vi "AILimits.vi"(0 "HighLimit":i16[](array[numeric])=[0, 0, 0, 0, 0, 0, 0, 0, 0, 0, 0, 0, 0, 0, 0, 0], 1 "ClearLimits":bool, 5 "LowLimit":i16[](array[numeric])=[0, 0, 0, 0, 0, 0, 0, 0, 0, 0, 0, 0, 0, 0, 0, 0], 7 "UnscaledAI":i16[](array[numeric])=[0, 0, 0, 0, 0, 0, 0, 0, 0, 0, 0, 0, 0, 0, 0, 0], 11 "index":i16, 12 "LimitsEnabled":u16 format="%.0x") -> (4 "UnscaledLimitLowOut":u16 format="%.0x", 6 "UnscaledLimitHighOut":u16 format="%.0x")   [LabVIEW 2017, in "ScaleAndLimit.lvlib"]
uses:
  ScaleAndLimit.lvlib
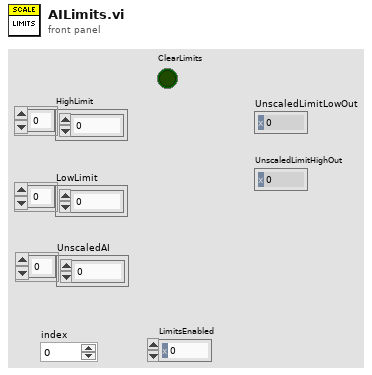
[diagram p1: front panel]
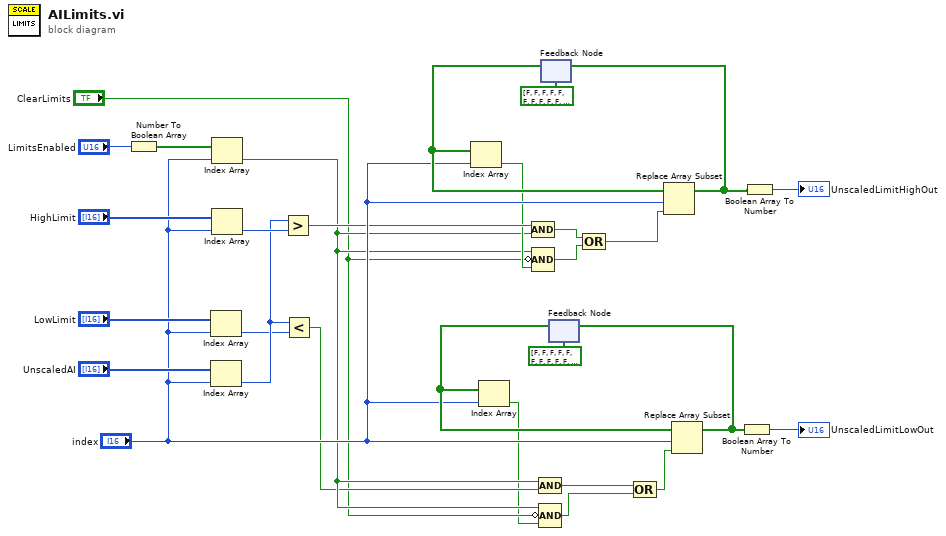
[diagram p0: block diagram]
diagram:
  n1 = Number To Boolean Array(number="LimitsEnabled") -> (Boolean array=w22:bool[])
  n2 = Index Array(array="LowLimit", index="index") -> (element=w24:i16)
  n3 = Index Array(array="UnscaledAI", index="index") -> (element=w25:i16)
  n4 = Index Array(array=w22, index="index") -> (element=w6:bool)
  n5 = Index Array(array="HighLimit", index="index") -> (element=w26:i16)
  n6 = Greater?(x=w25, y=w26) -> (0:w11:bool)
  n7 = Less?(x=w25, y=w24) -> (x < y?=w5:bool)
  n8 = Compound Arithmetic op=AND(w11, w6) -> (w9:bool)
  n9 = Compound Arithmetic op=AND(w6, w5) -> (w2:bool)
  n10 = feedback #1(bool[] [FALSE, FALSE, FALSE, FALSE, FALSE, FALSE, FALSE, FALSE, FALSE, FALSE, FALSE, FALSE, FALSE, FALSE, FALSE, FALSE]) -> (w20:bool[])
  n11 = Index Array(array=w20, index="index") -> (element=w10:bool)
  n12 = Compound Arithmetic op=AND(w6, invert "ClearLimits", w10) -> (w8:bool)
  n13 = feedback #2(bool[] [FALSE, FALSE, FALSE, FALSE, FALSE, FALSE, FALSE, FALSE, FALSE, FALSE, FALSE, FALSE, FALSE, FALSE, FALSE, FALSE]) -> (w18:bool[])
  n14 = Index Array(array=w18, index="index") -> (element=w3:bool)
  n15 = Compound Arithmetic op=AND(w6, invert "ClearLimits", w3) -> (w1:bool)
  n16 = Compound Arithmetic op=OR(w9, w8) -> (w7:bool)
  n17 = Compound Arithmetic op=OR(w2, w1) -> (w19:bool)
  n18 = Replace Array Subset(array=w20, new element=w7, index="index") -> (w15:bool[])
  n19 = feedback-in #1(w15) -> ()
  n20 = Replace Array Subset(array=w18, new element=w19, index="index") -> (w13:bool[])
  n21 = feedback-in #2(w13) -> ()
  n22 = Boolean Array To Number(Boolean array=w13) -> (number=→"UnscaledLimitLowOut":u16)
  n23 = Boolean Array To Number(Boolean array=w15) -> (number=→"UnscaledLimitHighOut":u16)
